vi "ShooterSetup.vi"(11 "output cluster":T1) -> ()   [LabVIEW 2013]
uses:
  Events.vi
  ButtonLayoutOpJoyReg.ctl
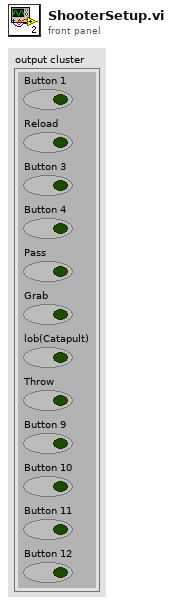
[diagram p1: front panel]
types:
  T1 = typedef "ButtonLayoutOpJoyReg.ctl" = cluster{"Button 1":bool, "Reload":bool, "Button 3":bool, "Button 4":bool, "Pass":bool, "Grab":bool, "lob(Catapult)":bool, "Throw":bool, "Button 9":bool, "Button 10":bool, "Button 11":bool, "Button 12":bool}
  T2 = cluster{"Reloading?":bool, "Throw":bool, "Ready?":bool, "Lob":bool, "Power":bool}
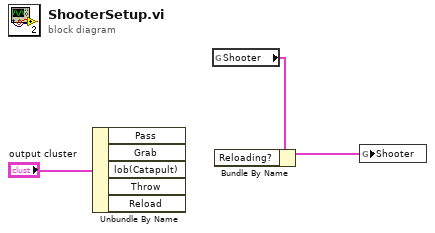
[diagram p0: block diagram]
diagram:
  n1 = Unbundle By Name("output cluster") -> ()  [unwired: 5 out]
  n2 = global read "Events.vi" "Shooter"() -> (w1:T2)
  n3 = Bundle By Name(cluster=w1) -> (w2:T2)  [unwired: 1 in]
  n4 = global write "Events.vi" "Shooter"(w2) -> ()
